vi "ConfigureMQTT.vi"(8 "error in (no error)":errorcluster, 10 "base path":path, 11 "Module ID":i32) -> (0 "error out":errorcluster, 2 "Subscriptions":variant, 3 "broadcasts":variant)   [LabVIEW 2015]
uses:
  Libraries/MQTT.lvlibp
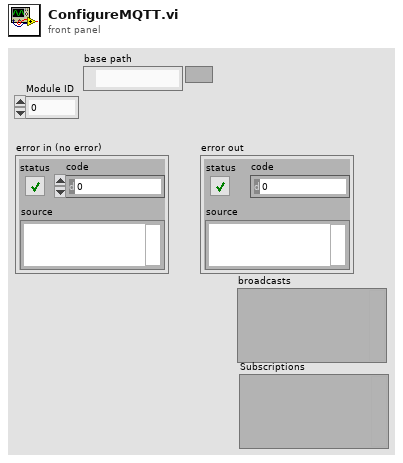
[diagram p1: front panel]
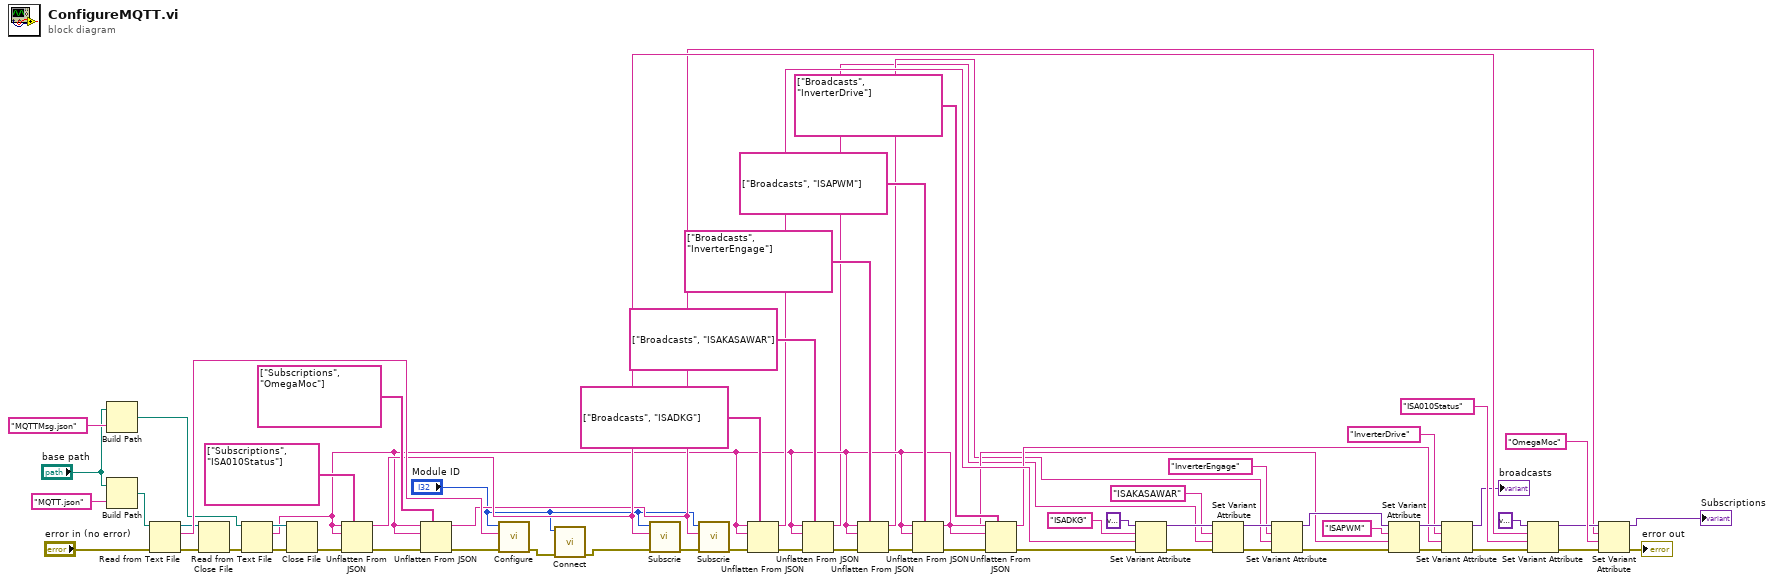
[diagram p0: block diagram]
diagram:
  n1 = Build Path(base path="base path", name or relative path="MQTTMsg.json") -> (appended path=w45:path)
  n2 = Build Path(base path="base path", name or relative path="MQTT.json") -> (appended path=w42:path)
  n3 = Read from Text File(file (use dialog)=w42, error in="error in (no error)") -> (refnum out=w41:refnum<file>, text=w48:string, error out=w43:errorcluster)  [unwired: 2 in, 1 out]
  n4 = Close File(refnum=w41, error in=w43) -> (error out=w46:errorcluster)  [unwired: 1 out]
  n5 = Read from Text File(file (use dialog)=w45, error in=w46) -> (refnum out=w47:refnum<file>, text=w30:string, error out=w44:errorcluster)  [unwired: 2 in, 1 out]
  n6 = Close File(refnum=w47, error in=w44) -> (error out=w34:errorcluster)  [unwired: 1 out]
  n7 = Unflatten From JSON(path=string[] ["Subscriptions", "ISA010Status"], JSON string=w30, type and defaults=w30, error in (no error)=w34) -> (value=w36:string, error out=w54:errorcluster)  [unwired: 3 in]
  n8 = Unflatten From JSON(path=string[] ["Subscriptions", "OmegaMoc"], JSON string=w30, type and defaults=w30, error in (no error)=w54) -> (value=w35:string, error out=w5:errorcluster)  [unwired: 3 in]
  n9 = call "Configure.vi"("error in (no error)"=w5, "JSON config"=w48, "Module ID"="Module ID") -> ("error out"=w3:errorcluster)  [unwired: 8 in]
  n10 = call "Connect.vi"("error in (no error)"=w3, "Module ID"="Module ID") -> ("error out"=w2:errorcluster)  [unwired: 9 in]
  n11 = call "Subscrie.vi"("error in (no error)"=w2, "String"=w36, "Module ID"="Module ID") -> ("error out"=w38:errorcluster)  [unwired: 8 in]
  n12 = call "Subscrie.vi"("error in (no error)"=w38, "String"=w35, "Module ID"="Module ID") -> ("error out"=w4:errorcluster)  [unwired: 8 in]
  n13 = Unflatten From JSON(path=string[] ["Broadcasts", "ISADKG"], JSON string=w30, type and defaults=w30, error in (no error)=w4) -> (value=w31:string, error out=w17:errorcluster)  [unwired: 3 in]
  n14 = Unflatten From JSON(path=string[] ["Broadcasts", "ISAKASAWAR"], JSON string=w30, type and defaults=w30, error in (no error)=w17) -> (value=w18:string, error out=w16:errorcluster)  [unwired: 3 in]
  n15 = Unflatten From JSON(path=string[] ["Broadcasts", "InverterEngage"], JSON string=w30, type and defaults=w30, error in (no error)=w16) -> (value=w19:string, error out=w15:errorcluster)  [unwired: 3 in]
  n16 = Unflatten From JSON(path=string[] ["Broadcasts", "ISAPWM"], JSON string=w30, type and defaults=w30, error in (no error)=w15) -> (value=w20:string, error out=w10:errorcluster)  [unwired: 3 in]
  n17 = Unflatten From JSON(path=string[] ["Broadcasts", "InverterDrive"], JSON string=w30, type and defaults=w30, error in (no error)=w10) -> (value=w21:string, error out=w9:errorcluster)  [unwired: 3 in]
  n18 = Set Variant Attribute(Variant=variant ("variant"), name="ISADKG", value=w31, error in=w9) -> (Variant out=w29:variant, error out=w14:errorcluster)  [unwired: 1 out]
  n19 = Set Variant Attribute(Variant=w29, name="ISAKASAWAR", value=w18, error in=w14) -> (Variant out=w28:variant, error out=w13:errorcluster)  [unwired: 1 out]
  n20 = Set Variant Attribute(Variant=w28, name="InverterEngage", value=w19, error in=w13) -> (Variant out=w27:variant, error out=w12:errorcluster)  [unwired: 1 out]
  n21 = Set Variant Attribute(Variant=w27, name="ISAPWM", value=w20, error in=w12) -> (Variant out=w26:variant, error out=w11:errorcluster)  [unwired: 1 out]
  n22 = Set Variant Attribute(Variant=w26, name="InverterDrive", value=w21, error in=w11) -> (Variant out=→"broadcasts":variant, error out=w8:errorcluster)  [unwired: 1 out]
  n23 = Set Variant Attribute(Variant=variant ("variant"), name=w36, value="ISA010Status", error in=w8) -> (Variant out=w56:variant, error out=w55:errorcluster)  [unwired: 1 out]
  n24 = Set Variant Attribute(Variant=w56, name=w35, value="OmegaMoc", error in=w55) -> (Variant out=→"Subscriptions":variant, error out=→"error out":errorcluster)  [unwired: 1 out]
